vi "关闭子VI.vi"(8 "错误输入":errorcluster caption="错误输入（无错误）", 11 "引用":refnum<vi>) -> (0 "错误输出":errorcluster, 3 "引用输出":refnum<vi>)   [LabVIEW 2018]
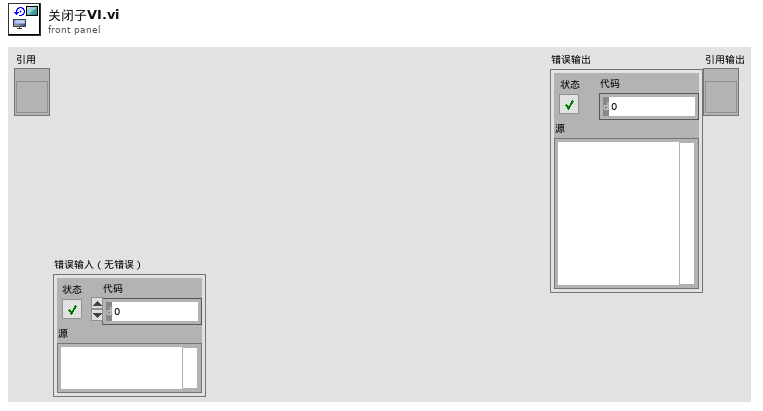
[diagram p1: front panel]
types:
  T1 = enum32{"Invalid", "Standard", "Closed", "Hidden", "Minimized", "Maximized"}
  T2 = enum32{"Bad", "Idle", "Run top level", "Running"}
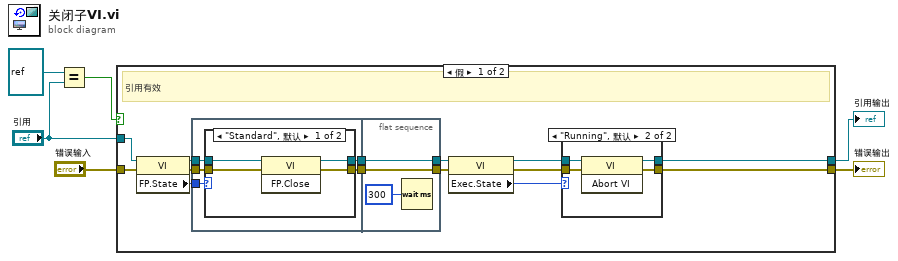
[diagram p0: block diagram]
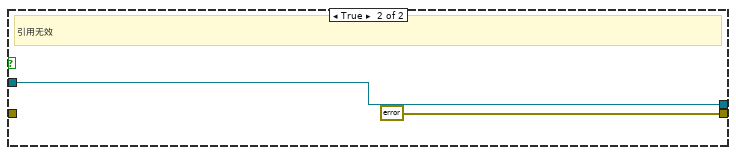
[diagram p4: hidden frame]
diagram:
  n1 = Equal?(x=refnum<vi> refnum ("引用"), y="引用") -> (x = y?=w5:bool)
  n2 = case shown="假" w5 {
    tunnel: [w9 errorcluster {"status"=FALSE, "code"=0, "source"=""} ("error out")] -> w1
    tunnel: "错误输入" -> [w16 _]
    tunnel: [w10 w42] -> w2
    tunnel: "引用" -> [w17 w42]
    frame False {
      # "引用有效"
      n3 = property class="VI"(reference=w17, error in=w16) -> (reference out=w20:refnum<vi>, error out=w18:errorcluster, "FP.State"=w19:T1)
      n4 = flat-sequence {
        tunnel: w20 -> [w25]
        tunnel: w19 -> [w24]
        tunnel: w18 -> [w23]
        tunnel: [w22] -> w8
        tunnel: [w21] -> w7
        tunnel: [w33] -> w11
        tunnel: [w34] -> w12
        tunnel: w8 -> [w34]
        tunnel: w7 -> [w33]
        frame #0 {
          n5 = case shown="\"Standard\", 默认" w24 {
            tunnel: [w28 w31] -> w22
            tunnel: [w27 w30] -> w21
            tunnel: w25 -> [w29 w31]
            tunnel: w23 -> [w26 w30]
            frame "Standard", Default {
              n6 = invoke class="VI" method="FP.Close"(reference=w29, error in=w26) -> (reference out=w28:refnum<vi>, error out=w27:errorcluster)  [unwired: 1 in, 1 out]
            }
            frame "Invalid", "Closed" {
            }
          }
        }
        frame #1 {
          n7 = Wait (ms)(milliseconds to wait=u32 300 ("等待时间（毫秒）")) -> ()  [unwired: 1 out]
        }
      }
      n8 = property class="VI"(reference=w12, error in=w11) -> (reference out=w15:refnum<vi>, error out=w13:errorcluster, "Exec.State"=w14:T2)
      n9 = case shown="\"Running\", 默认" w14 {
        tunnel: [w36 w38] -> w10
        tunnel: [w35 w37] -> w9
        tunnel: w15 -> [w36 w40]
        tunnel: w13 -> [w35 w39]
        frame "Idle" {
        }
        frame "Running", Default {
          n10 = invoke class="VI" method="Abort VI"(reference=w40, error in=w39) -> (reference out=w38:refnum<vi>, error out=w37:errorcluster)  [unwired: 1 in, 1 out]
        }
      }
    }
    frame True {
      # "引用无效"
    }
  }
  "错误输出" <- w1
  "引用输出" <- w2
